vi "Serial.vi"(2 "error in (no error)":errorcluster caption="错误输入（无错误）", 3 "串口设置":T1={"波特率"=115200, "数据位"=8, "校验"=enum."None", "停止位"=10, "VISA资源名称"="COM1", "XON"=enum."DC1", "XOFF"=enum."DC3", "终止符时结束读取？"=TRUE, "终止符"=10, "流控制"=0} {"流控制" items=["无"=0, "XON/XOFF"=1, "RTS/CTS"=2, "DTR/DSR"=4]; "终止符" format="%.0x"; "停止位" items=["1.0"=10, "1.5"=15, "2.0"=20]; "数据位" min=5 max=8 step=1; "波特率" items=["75"=75, "110"=110, "134"=134, "150"=150, "300"=300, "600"=600, "1200"=1200, "1800"=1800, "2400"=2400, "4800"=4800, "7200"=7200, "9600"=9600, "14400"=14400, "19200"=19200, "28800"=28800, "38400"=38400, "56000"=56000, "57600"=57600, "115200"=115200, "128000"=128000, "230400"=230400]}) -> (0 "错误输出":errorcluster, 1 "VISA resource name out":refnum<visa-resource-name>)   [LabVIEW 2019]
uses:
  <vilib>/Instr/_visa.llb/VISA Configure Serial Port (Instr).vi
panel:
  # "IN"
  # "OUT"
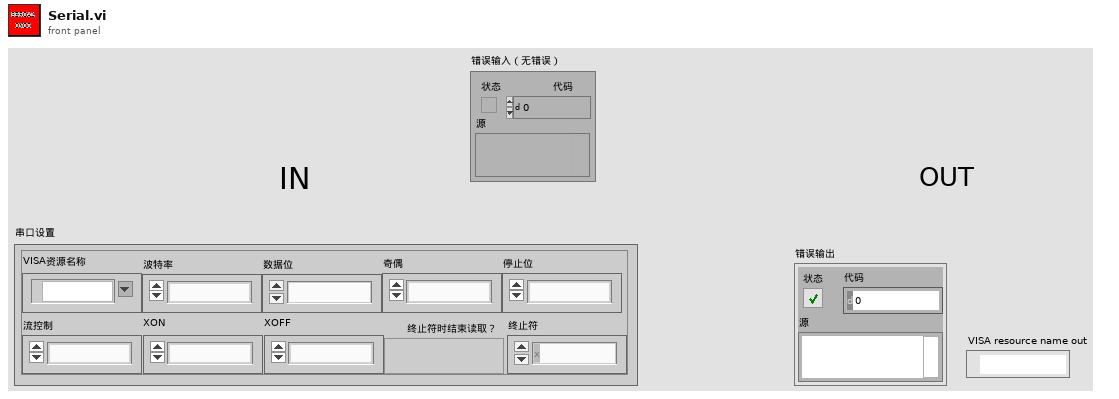
[diagram p1: front panel]
types:
  T1 = cluster{"波特率":u32, "数据位":u16, "校验":enum16{"None", "Odd", "Even", "Mark", "Space"}, "停止位":u16, "VISA资源名称":refnum<visa-resource-name>, "XON":enum16{"NUL", "SOH", "STX", "ETX", "EOT", "ENQ", "ACK", "BEL", "BS", "HT", "LF", "VT", "FF", "CR", "SO", "SI", "DLE", "DC1", "DC2", "DC3", "DC4", "NAK", "SYN", "ETB", "CAN", "EM", "SUB", "ESC", "FS", "GS", "RS", "US", "SP", "!", "\"", "#", "$", "%", "&", "'", "(", ")", "*", "+", ",", "- (-)", ".", "/", "0", "1", "2", "3", "4", "5", "6", "7", "8", "9", ":", ";", "<", "=", ">", "?", "@", "A", "B", "C", "D", "E", "F", "G", "H", "I", "J", "K", "L", "M", "N", "O", "P", "Q", "R", "S", "T", "U", "V", "W", "X", "Y", "Z", "[", "\\", "]", "^", "_", "`", "a", "b", "c", "d", "e", "f", "g", "h", "i", "j", "k", "l", "m", "n", "o", "p", "q", "r", "s", "t", "u", "v", "w", "x", "y", "z", "{", "|", "}", "~"}, "XOFF":enum16{"NUL", "SOH", "STX", "ETX", "EOT", "ENQ", "ACK", "BEL", "BS", "HT", "LF", "VT", "FF", "CR", "SO", "SI", "DLE", "DC1", "DC2", "DC3", "DC4", "NAK", "SYN", "ETB", "CAN", "EM", "SUB", "ESC", "FS", "GS", "RS", "US", "SP", "!", "\"", "#", "$", "%", "&", "'", "(", ")", "*", "+", ",", "- (-)", ".", "/", "0", "1", "2", "3", "4", "5", "6", "7", "8", "9", ":", ";", "<", "=", ">", "?", "@", "A", "B", "C", "D", "E", "F", "G", "H", "I", "J", "K", "L", "M", "N", "O", "P", "Q", "R", "S", "T", "U", "V", "W", "X", "Y", "Z", "[", "\\", "]", "^", "_", "`", "a", "b", "c", "d", "e", "f", "g", "h", "i", "j", "k", "l", "m", "n", "o", "p", "q", "r", "s", "t", "u", "v", "w", "x", "y", "z", "{", "|", "}", "~"}, "终止符时结束读取？":bool, "终止符":u8, "流控制":u16}
  T2 = enum16{"NUL", "SOH", "STX", "ETX", "EOT", "ENQ", "ACK", "BEL", "BS", "HT", "LF", "VT", "FF", "CR", "SO", "SI", "DLE", "DC1", "DC2", "DC3", "DC4", "NAK", "SYN", "ETB", "CAN", "EM", "SUB", "ESC", "FS", "GS", "RS", "US", "SP", "!", "\"", "#", "$", "%", "&", "'", "(", ")", "*", "+", ",", "- (-)", ".", "/", "0", "1", "2", "3", "4", "5", "6", "7", "8", "9", ":", ";", "<", "=", ">", "?", "@", "A", "B", "C", "D", "E", "F", "G", "H", "I", "J", "K", "L", "M", "N", "O", "P", "Q", "R", "S", "T", "U", "V", "W", "X", "Y", "Z", "[", "\\", "]", "^", "_", "`", "a", "b", "c", "d", "e", "f", "g", "h", "i", "j", "k", "l", "m", "n", "o", "p", "q", "r", "s", "t", "u", "v", "w", "x", "y", "z", "{", "|", "}", "~"}
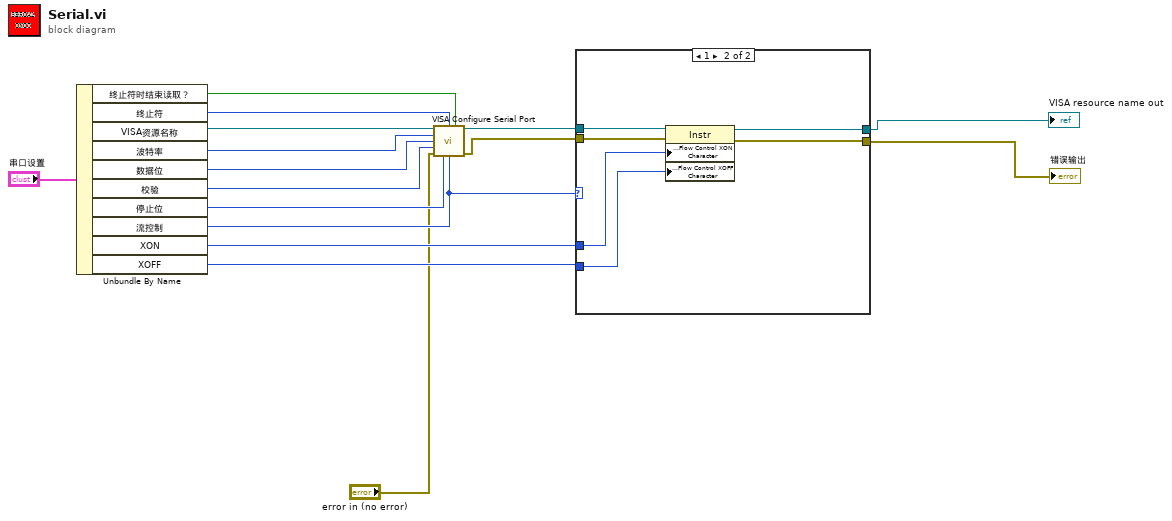
[diagram p0: block diagram]
diagram:
  n1 = Unbundle By Name("串口设置") -> ("终止符时结束读取？"=w4:bool, "终止符"=w3:u8, "VISA资源名称"=w5:refnum<visa-resource-name>, "波特率"=w6:u32, "数据位"=w7:u16, "校验"=w8:enum16{"None", "Odd", "Even", "Mark", "Space"}, "停止位"=w9:u16, "流控制"=w2:u16, "XON"=w11:T2, "XOFF"=w10:T2)
  n2 = call-poly "VISA Configure Serial Port"("VISA resource name"=w5, "termination char\n(0xA = '\\n' = LF)"=w3, "Enable Termination\nChar (T)"=w4, "baud rate (9600)"=w6, "data bits (8)"=w7, "parity (0:none)"=w8, "error in (no error)"="error in (no error)", "stop bits (10: 1 bit)"=w9, "flow control (0:none)"=w2) -> ("VISA resource name out"=w15:refnum<visa-resource-name>, "error out"=w14:errorcluster)  [unwired: 1 in, 4 out]
  n3 = case shown="1" w2 {
    tunnel: [w17 w24] -> w12
    tunnel: [w18 w23] -> w13
    tunnel: w15 -> [w18 w22]
    tunnel: w14 -> [w17 w21]
    tunnel: w11 -> [_ w20]
    tunnel: w10 -> [_ w19]
    frame Default {
    }
    frame 1 {
      n4 = property class="Instr"(reference=w22, error in=w21, "Serial Settings:Flow Control XON Character"=w20, "Serial Settings:Flow Control XOFF Character"=w19) -> (reference out=w23:refnum<visa-resource-name>, error out=w24:errorcluster)
    }
  }
  "错误输出" <- w12
  "VISA resource name out" <- w13
